vi "CODCr微站质控流程 (子VI).vi"(10 "CODCr量程切换":enum32{"H", "L", "AUTO"}(ring)=enum."AUTO", 11 "CODCr":bool) -> (2 "CODCr中断报警":bool, 3 "布尔":bool)   [LabVIEW 2016, in "质控单元.lvlib"]
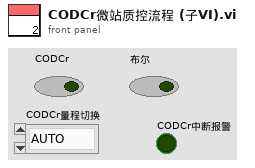
[diagram p1: front panel]
types:
  T1 = enum16{"待机", "启动水样测量", "水样测量中", "启动加标", "启动加标回收", "加标回收测量中", "结束"}
  T2 = cluster{"测量模式":enum16{"水样测量", "标样核查", "零点核查", "跨度核查", "空白测试", "加标回收", "平行样", "校零", "校标"}}
  T3 = enum16{"空闲", "水样测试", "标样核查", "零点核查", "跨度核查", "空白测试", "平行样测试", "加标回收", "空白校准", "标样校准", "初始化（清洗）"}
  T4 = cluster{"系统时间":timestamp, "工作状态":enum16{"空闲", "水样测试", "标样核查", "零点核查", "跨度核查", "空白测试", "平行样测试", "加标回收", "空白校准", "标样校准", "初始化（清洗）"}, "测量模式":enum16{"待机", "连续模式", "周期模式", "定点模式", "受控模式", "手动模式"}, "告警代码":enum16{"无告警", "缺试剂告警", "缺水样告警", "缺蒸馏水告警", "缺标液告警", "仪表漏液告警", "标定异常告警", "超量程告警", "加热异常", "低试剂预警", "超上限告警", "超下限告警", "仪表内部其他异常", "滴定异常告警", "电极异常告警", "量程切换告警", "参数设置告警", "PH电极电位异常", "电导率电极异常", "浊度光度异常", "溶解氧电极异常", "溶解氧光强异常", "温度异常告警", "PH异常告警", "溶解氧异常告警", "电导率异常告警", "浊度异常告警", "叶绿素异常告警", "藻密度异常告警", "蓝绿藻异常告警", "ORP异常告警", "氨氮异常告警", "清洁刷异常告警", "SD卡异常告警", "蓝牙异常告警", "Wifi异常告警", "流程异常告警"}, "故障代码":enum16{"无故障", "电机故障", "温度故障", "通讯故障", "滴定故障"}, "日志代码":u16, "软件版本":u16, "F0":sgl, "F1":sgl, "F2":sgl, "F3":sgl, "T":sgl, "H":sgl, "id":u16, "flowid":u16, "量程":u16, "总磷控温温度1":sgl, "营养盐控温温度2":sgl, "ADC":sgl}
  T5 = cluster{"因子编码":u32, "单位":u16, "标样参考值":sgl, "水样数据时间":timestamp, "水样实测值":sgl, "水样数据标识":string, "标样数据时间":timestamp, "标样实测值":sgl, "标样数据标识":string, "空白数据时间":timestamp, "空白实测值":sgl, "空白数据标识":string, "零点核查数据时间":timestamp, "零点核查实测值":sgl, "零点核查数据标识":string, "跨度核查数据时间":timestamp, "跨度核查实测值":sgl, "跨度核查数据标识":string, "加标回收数据时间":timestamp, "加标回收实测值":sgl, "加标回收数据标识":string, "平行样数据时间":timestamp, "平行样实测值":sgl, "平行样数据标识":string}
  T6 = cluster{"量程":dbl, "检出限":dbl, "加标前水样浓度":dbl, "加标后水样浓度":dbl, "加标水杯定容体积":dbl, "加标母液浓度":dbl, "加标体积":dbl, "加标回收率":dbl}
  T7 = cluster{"氨氮":u8, "总磷":u8, "总氮":u8, "CODMn":u8, "CODCr":u8}
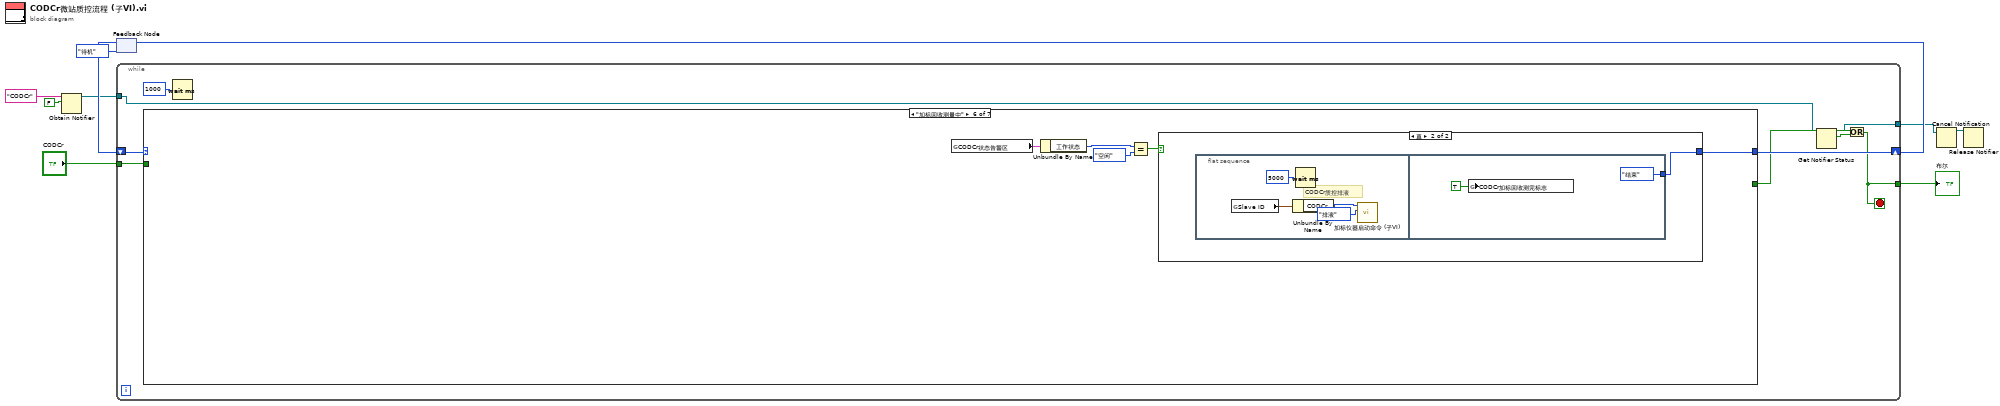
[diagram p0: block diagram]
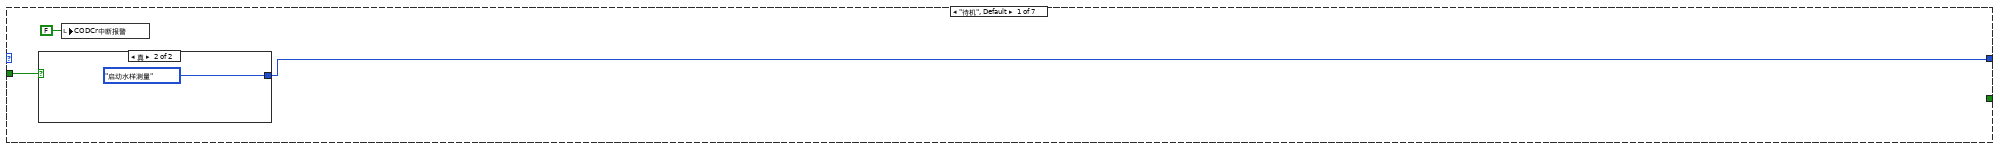
[diagram p2: hidden frame]
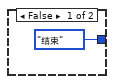
[diagram p3: hidden frame]
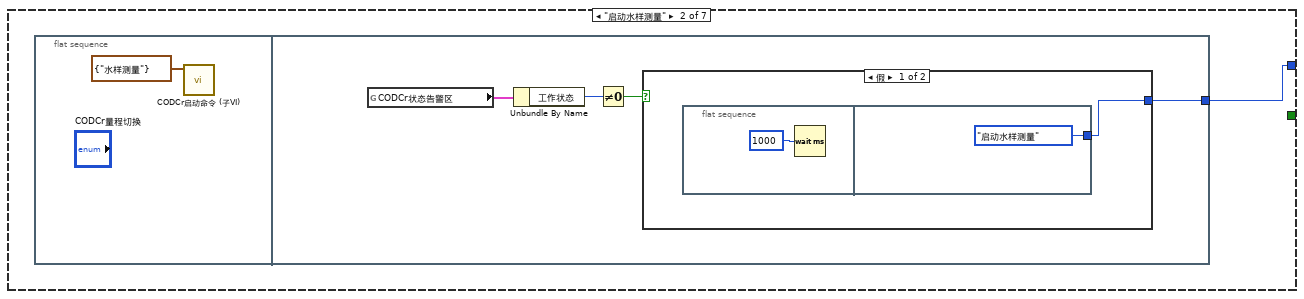
[diagram p4: hidden frame]
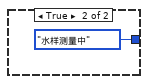
[diagram p5: hidden frame]
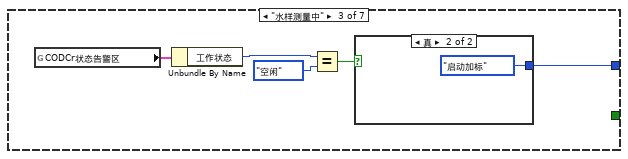
[diagram p6: hidden frame]
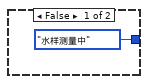
[diagram p7: hidden frame]
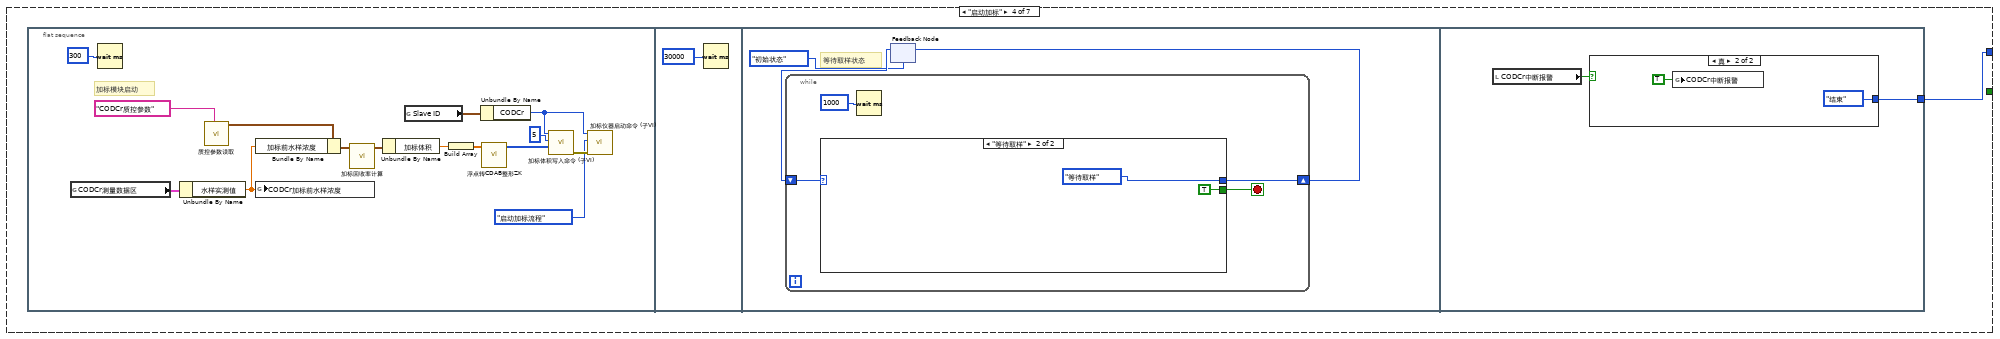
[diagram p8: hidden frame]
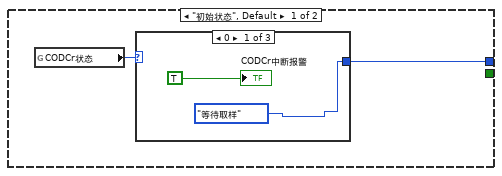
[diagram p9: hidden frame]
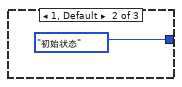
[diagram p10: hidden frame]
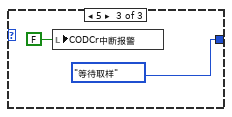
[diagram p11: hidden frame]
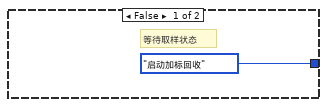
[diagram p12: hidden frame]
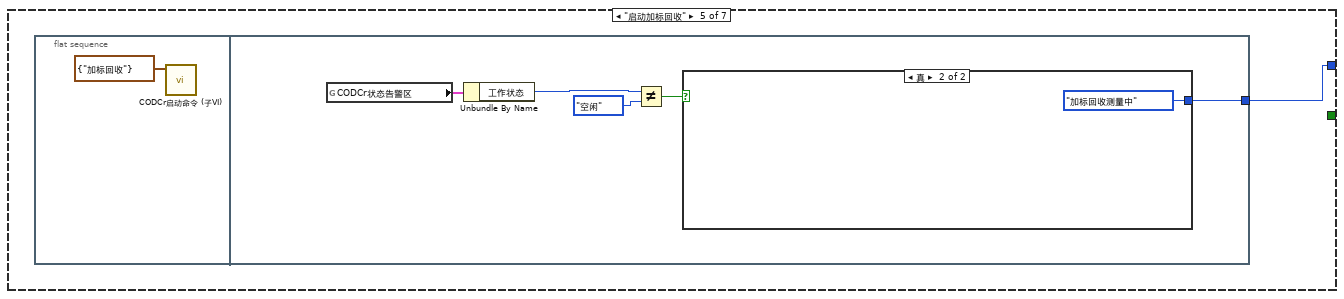
[diagram p13: hidden frame]
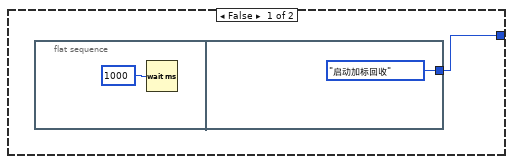
[diagram p14: hidden frame]
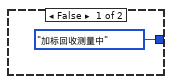
[diagram p15: hidden frame]
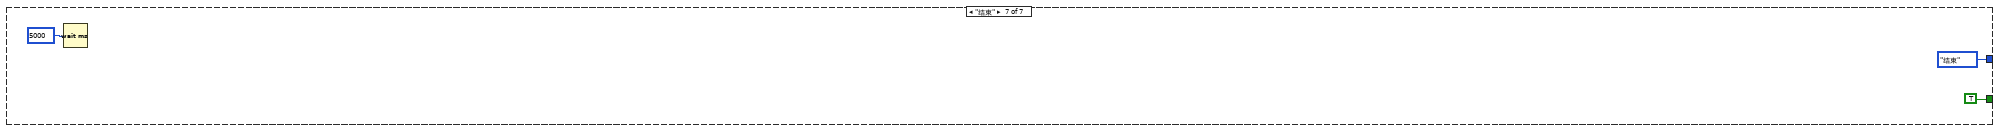
[diagram p16: hidden frame]
diagram:
  n1 = Obtain Notifier(name (unnamed)="CODCr" ("名称（未命名）"), notification data type=FALSE) -> (notifier out=w3:refnum<notifier>)  [unwired: 2 in, 2 out]
  n2 = feedback #1(T1."待机") -> (w6:T1)
  n3 = while {
    tunnel: "CODCr" -> [w19]
    tunnel: [w14] -> w8
    shift-right: [w18] -> w9
    shift-left: w6 -> [w17]
    tunnel: w3 -> [w12]
    tunnel: [w11] -> w1
    stop <- w14 stop-if-true
    n4 = case shown="\"加标回收测量中\"" w17 {
      tunnel: [w22 w25 w39 w42 w80 w95 T1."结束"] -> w18
      tunnel: [_ _ _ _ _ _ TRUE] -> w13
      tunnel: w19 -> [w21 _ _ _ _ _ _]
      frame "待机", Default {
        n5 = case shown="真" w21 {
          tunnel: [T1."结束" T1."启动水样测量"] -> w22
          frame False {
          }
          frame True {
          }
        }
        n6 = local write "CODCr中断报警"(FALSE ("CODMn中断报警")) -> ()
      }
      frame "启动水样测量" {
        n7 = flat-sequence {
          tunnel: [w30] -> w25
          frame #0 {
            n8 = call "CODCr启动命令 (子VI).vi"("启动测量模式"=T2 {"测量模式"=enum."水样测量"}) -> ()  [unwired: 10 in, 1 out]
          }
          frame #1 {
            n9 = global read "与CODCr交互全局.vi" "CODCr状态告警区"() -> (w28:T4)
            n10 = Unbundle By Name(w28) -> ("工作状态"=w29:T3)
            n11 = Not Equal To 0?(x=w29) -> (x != 0?=w27:bool)
            n12 = case shown="假" w27 {
              tunnel: [w31 T1."水样测量中"] -> w30
              frame False {
                n13 = flat-sequence {
                  tunnel: [T1."启动水样测量"] -> w31
                  frame #0 {
                    n14 = Wait (ms)(milliseconds to wait=u32 1000 ("等待时间（毫秒）")) -> ()  [unwired: 1 out]
                  }
                  frame #1 {
                  }
                }
              }
              frame True {
              }
            }
          }
        }
      }
      frame "水样测量中" {
        n15 = global read "与CODCr交互全局.vi" "CODCr状态告警区"() -> (w36:T4)
        n16 = Unbundle By Name(w36) -> ("工作状态"=w35:T3)
        n17 = Equal?(x=w35, y=T3."空闲") -> (x = y?=w37:bool)
        n18 = case shown="真" w37 {
          tunnel: [T1."水样测量中" T1."启动加标"] -> w39
          frame False {
          }
          frame True {
          }
        }
      }
      frame "启动加标" {
        n19 = flat-sequence {
          tunnel: [w76] -> w42
          frame #0 {
            # "加标模块启动"
            n20 = global read "与CODCr交互全局.vi" "CODCr测量数据区"() -> (w49:T5)
            n21 = Wait (ms)(milliseconds to wait=u32 300 ("等待时间（毫秒）")) -> ()  [unwired: 1 out]
            n22 = Unbundle By Name(w49) -> ("水样实测值"=w50:sgl)
            n23 = call "质控参数读取.vi"("section"="CODCr质控参数") -> ("参数"=w55:T6)  [unwired: 9 in, 1 out]
            n24 = Bundle By Name(cluster=w55, "加标前水样浓度"=w50) -> (w56:T6)
            n25 = global write "水样浓度全局.vi" "CODCr加标前水样浓度"(w50) -> ()
            n26 = call "加标回收率计算.vi"("参数"=w56) -> ("参数 out"=w54:T6)  [unwired: 9 in, 1 out]
            n27 = Unbundle By Name(w54) -> ("加标体积"=w52:dbl)
            n28 = global read "断电保存全局.vi" "Slave ID"() -> (w44:T7)
            n29 = Build Array(w52) -> (w53:dbl[])
            n30 = Unbundle By Name(w44) -> ("CODCr"=w43:u8)
            n31 = call "浮点转CDAB整形ZK.vi"("浮点数"=w53) -> ("CDAB整形输出"=w45:u16[])  [unwired: 10 in]
            n32 = call "加标体积写入命令 (子VI).vi"("values"=w45, "starting address"=u16 5, "Slave ID"=w43) -> ("错误输出"=w48:errorcluster)  [unwired: 8 in]
            n33 = call "加标仪器启动命令 (子VI).vi"("错误输入（无错误）"=w48, "启动命令"=enum16{"启动水样流程", "启动加标流程", "排液", "停止"}."启动加标流程", "仪器"=w43) -> ()  [unwired: 8 in, 1 out]
          }
          frame #1 {
            n34 = Wait (ms)(milliseconds to wait=u32 30000 ("等待时间（毫秒）")) -> ()  [unwired: 1 out]
          }
          frame #2 {
            # "等待取样状态"
            n35 = feedback #2(enum16{"初始状态", "等待取样"}."初始状态") -> (w61:enum16{"初始状态", "等待取样"})
            n36 = while {
              shift-right: [w64] -> w60
              shift-left: w61 -> [w65]
              stop <- w63 stop-if-true
              n37 = case shown="\"等待取样\"" w65 {
                tunnel: [w67 enum16{"初始状态", "等待取样"}."等待取样"] -> w64
                tunnel: [_ TRUE] -> w63
                frame "初始状态", Default {
                  n38 = global read "加标回收状态全局变量.vi" "CODCr状态"() -> (w66:u16)
                  n39 = case shown="0" w66 {
                    tunnel: [enum16{"初始状态", "等待取样"}."等待取样" enum16{"初始状态", "等待取样"}."初始状态" enum16{"初始状态", "等待取样"}."等待取样"] -> w67
                    frame 0 {
                      "CODCr中断报警" <- TRUE ("CODMn中断报警")
                    }
                    frame 1, Default {
                    }
                    frame 5 {
                      n40 = local write "CODCr中断报警"(FALSE ("CODMn中断报警")) -> ()
                    }
                  }
                }
                frame "等待取样" {
                }
              }
              n41 = Wait (ms)(milliseconds to wait=u32 1000 ("等待时间（毫秒）")) -> ()  [unwired: 1 out]
            }
            n42 = feedback-in #2(w60) -> ()
          }
          frame #3 {
            n43 = local read "CODCr中断报警"() -> (w75:bool)
            n44 = case shown="真" w75 {
              tunnel: [T1."启动加标回收" T1."结束"] -> w76
              frame False {
                # "等待取样状态"
              }
              frame True {
                n45 = global write "质控中断报警全局.vi" "CODCr中断报警"(TRUE ("CODCr中断报警")) -> ()
              }
            }
          }
        }
      }
      frame "启动加标回收" {
        n46 = flat-sequence {
          tunnel: [w86] -> w80
          frame #0 {
            n47 = call "CODCr启动命令 (子VI).vi"("启动测量模式"=T2 {"测量模式"=enum."加标回收"}) -> ()  [unwired: 10 in, 1 out]
          }
          frame #1 {
            n48 = global read "与CODCr交互全局.vi" "CODCr状态告警区"() -> (w85:T4)
            n49 = Unbundle By Name(w85) -> ("工作状态"=w84:T3)
            n50 = Not Equal?(x=w84, y=T3."空闲") -> (x != y?=w82:bool)
            n51 = case shown="真" w82 {
              tunnel: [w87 T1."加标回收测量中"] -> w86
              frame False {
                n52 = flat-sequence {
                  tunnel: [T1."启动加标回收"] -> w87
                  frame #0 {
                    n53 = Wait (ms)(milliseconds to wait=u32 1000 ("等待时间（毫秒）")) -> ()  [unwired: 1 out]
                  }
                  frame #1 {
                  }
                }
              }
              frame True {
              }
            }
          }
        }
      }
      frame "加标回收测量中" {
        n54 = global read "与CODCr交互全局.vi" "CODCr状态告警区"() -> (w92:T4)
        n55 = Unbundle By Name(w92) -> ("工作状态"=w91:T3)
        n56 = Equal?(x=w91, y=T3."空闲") -> (x = y?=w93:bool)
        n57 = case shown="真" w93 {
          tunnel: [T1."加标回收测量中" w97] -> w95
          frame False {
          }
          frame True {
            n58 = flat-sequence {
              tunnel: [T1."结束"] -> w97
              frame #0 {
                # "CODCr质控排液"
                n59 = global read "断电保存全局.vi" "Slave ID"() -> (w99:T7)
                n60 = Unbundle By Name(w99) -> ("CODCr"=w100:u8)
                n61 = Wait (ms)(milliseconds to wait=u32 5000 ("等待时间（毫秒）")) -> ()  [unwired: 1 out]
                n62 = call "加标仪器启动命令 (子VI).vi"("启动命令"=enum16{"启动水样流程", "启动加标流程", "排液", "停止"}."排液", "仪器"=w100) -> ()  [unwired: 9 in, 1 out]
              }
              frame #1 {
                n63 = global write "质控测完标志全局 1.vi" "CODCr加标回收测完标志"(TRUE ("COD加标回收测完标志")) -> ()
              }
            }
          }
        }
      }
      frame "结束" {
        n64 = Wait (ms)(milliseconds to wait=u32 5000 ("等待时间（毫秒）")) -> ()  [unwired: 1 out]
      }
    }
    n65 = Wait (ms)(milliseconds to wait=u32 1000 ("等待时间（毫秒）")) -> ()  [unwired: 1 out]
    n66 = Get Notifier Status(notifier=w12) -> (notifier out=w11:refnum<notifier>, current notification=w15:bool)  [unwired: 1 in, 3 out]
    n67 = Or(x=w13, y=w15) -> (x .or. y?=w14:bool)
  }
  "布尔" <- w8
  n68 = feedback-in #1(w9) -> ()
  n69 = Cancel Notification(0:w1) -> (8:w2:refnum<notifier>)  [unwired: 1 in, 2 out]
  n70 = Release Notifier(notifier=w2) -> ()  [unwired: 2 in, 3 out]
